vi "固定站CODMn测量流程.vi"(11 "控制命令":u16(ring)=1 items=["启动测量"=1, "标样核查"=2, "零点核查"=3, "跨度核查"=4, "空白测试"=5, "平行样测试"=6, "加标回收"=7, "空白校准"=8, "标样校准"=9, "初始化（清洗）"=10, "停止测试"=11, "仪器重启"=12, "校时"=13, "模式设置"=14, "测量间隔设置"=15, "调试"=22, "填充管路"=30, "清洗管路"=31, "清洗反应杯"=32]) -> ()   [LabVIEW 2016, in "斯坦道CODMn新电路板.lvlib"]
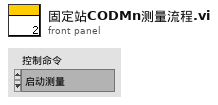
[diagram p1: front panel]
types:
  T1 = cluster{"仪器":enum16{"", "氨氮", "总磷", "总氮", "CODMn", "CODCr"}, "启动命令":enum16{"启动水样流程", "启动加标流程", "排液", "停止", "柱塞泵启动"}}
  T2 = cluster{"时间标识":timestamp, "设备":string, "日志信息":string, "备注":string}
  T3 = cluster{"站号":u16, "量程切换":enum32{"H", "L", "AUTO"}, "控制命令":u16, "模式设置":enum16{"待机", "连续模式", "周期模式", "定点模式", "受控模式", "手动模式"}, "测量间隔":u16}
  T4 = cluster{"系统时间":timestamp, "工作状态":u16, "测量模式":enum16{"待机", "连续模式", "周期模式", "定点模式", "受控模式", "手动模式"}, "告警代码":u16, "故障代码":u16, "日志代码":u16, "软件版本":u16, "A":sgl, "B":sgl, "K":sgl, "当前滴定数":sgl, "T":sgl, "H":sgl, "id":u16, "flowid":u16, "量程":u16, "加热实时温度":sgl, "当前ORP值":sgl, "运行时间":sgl, "当前步骤剩余时间":sgl, "结束滴定数":sgl, "注射泵保温温度":sgl}
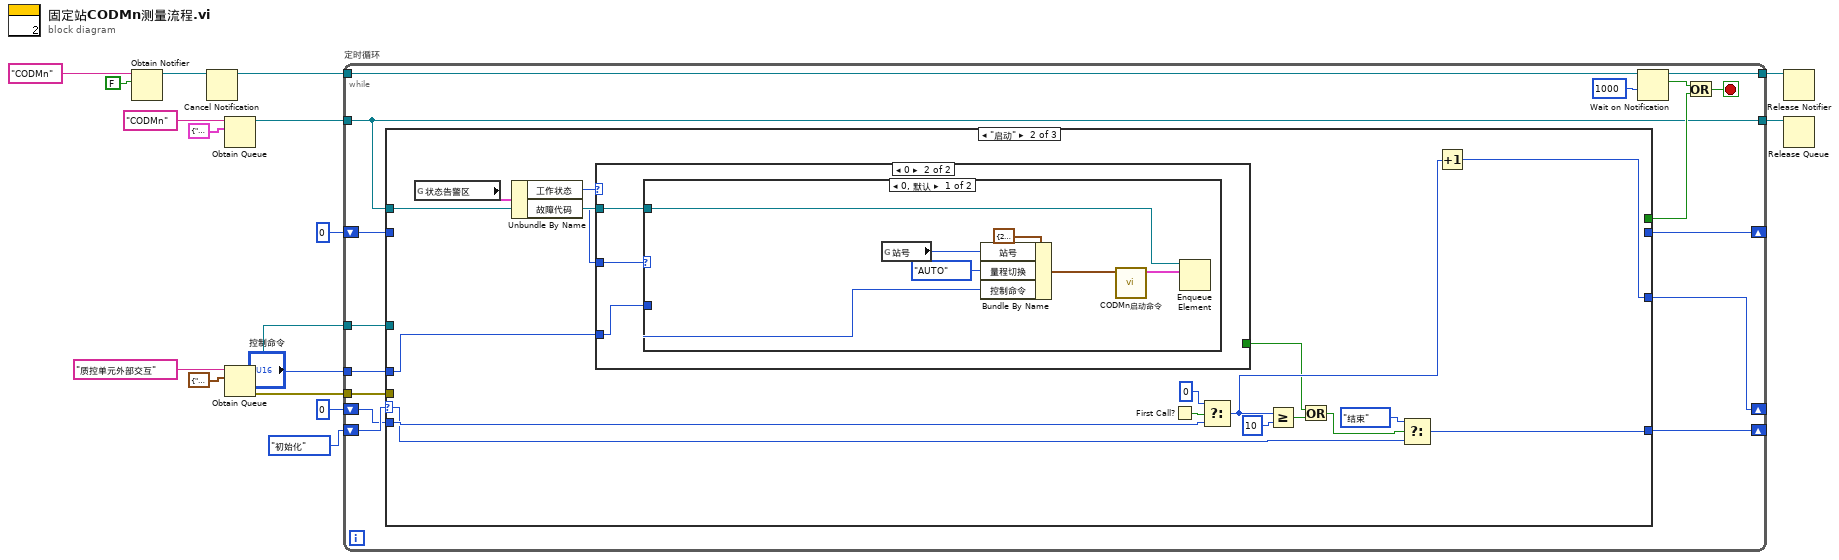
[diagram p0: block diagram]
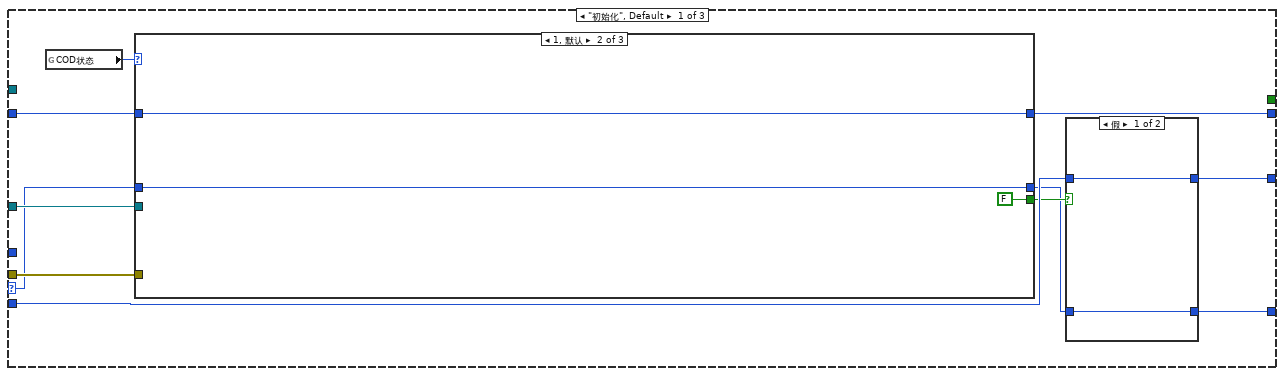
[diagram p2: hidden frame]
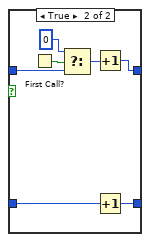
[diagram p3: hidden frame]
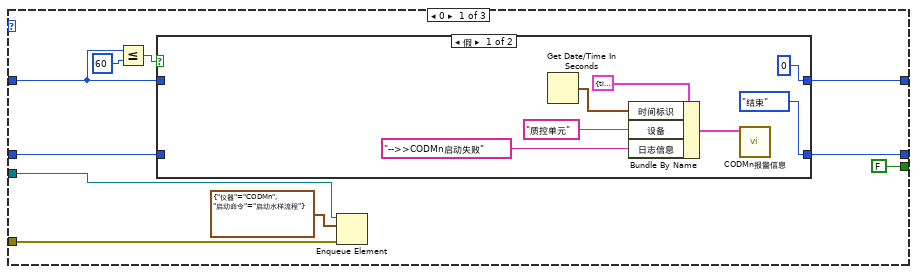
[diagram p4: hidden frame]
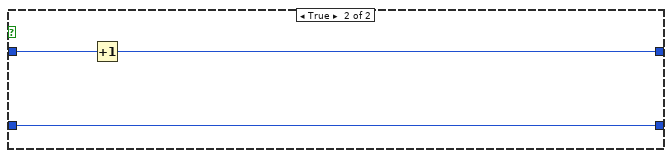
[diagram p5: hidden frame]
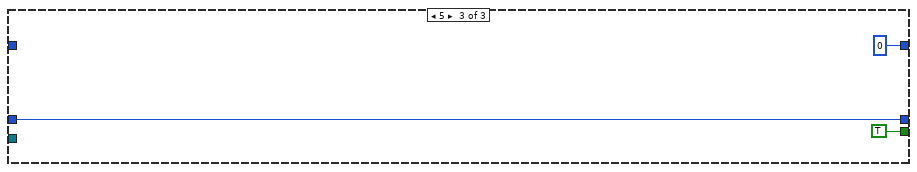
[diagram p6: hidden frame]
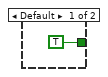
[diagram p7: hidden frame]
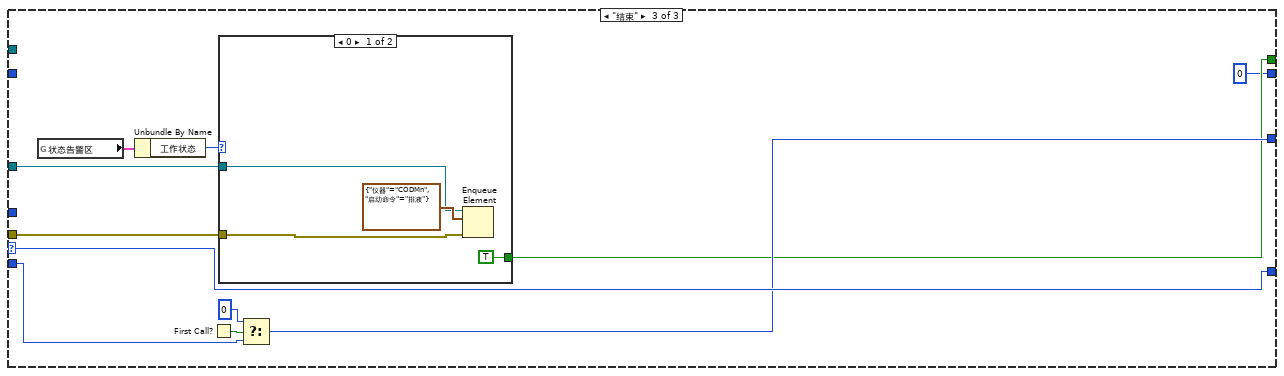
[diagram p9: hidden frame]
diagram:
  n1 = Obtain Notifier(name (unnamed)="CODMn" ("名称（未命名）"), notification data type=FALSE) -> (notifier out=w12:refnum<notifier>)  [unwired: 2 in, 2 out]
  n2 = Cancel Notification(0:w12) -> (8:w11:refnum<notifier>)  [unwired: 1 in, 2 out]
  n3 = Obtain Queue(name (unnamed)="CODMn" ("名称（未命名）"), element data type=cluster{"命令":string, "data":variant} {"命令"="", "data"=variant}) -> (queue out=w15:refnum<queue>)  [unwired: 3 in, 2 out]
  n4 = Obtain Queue(name (unnamed)="质控单元外部交互" ("名称（未命名）"), element data type=T1 {"仪器"=enum."氨氮", "启动命令"=enum."启动水样流程"} ("元素")) -> (queue out=w4:refnum<queue>, error out=w3:errorcluster)  [unwired: 3 in, 1 out]
  n5 = while "定时循环" {
    tunnel: w15 -> [w22]
    tunnel: w11 -> [w33]
    tunnel: "控制命令" -> [w28]
    shift-right: [w27] -> _
    shift-left: enum16{"初始化", "启动", "结束"}."初始化" -> [w29]
    shift-right: [w25] -> _
    shift-left: 0 -> [w26]
    tunnel: [w23] -> w7
    tunnel: [w22] -> w8
    tunnel: w4 -> [w21]
    tunnel: w3 -> [w20]
    shift-right: [w18] -> _
    shift-left: 0 -> [w19]
    stop <- w30 stop-if-true
    n6 = case shown="\"启动\"" w29 {
      selector: w29 -> [w35 w85 w118]
      tunnel: w28 -> [_ w96 _]
      tunnel: w22 -> [_ w95 _]
      tunnel: [w44 w86 w118] -> w27
      tunnel: w26 -> [w43 w90 w115]
      tunnel: [w42 w89 w114] -> w25
      tunnel: [_ _ w109] -> w24
      tunnel: w21 -> [w39 _ w113]
      tunnel: w20 -> [w38 _ w112]
      tunnel: w19 -> [w37 _ _]
      tunnel: [w36 _ 0] -> w18
      frame "初始化", Default {
        n7 = global read "VARCODMn全局变量.vi" "COD状态"() -> (w40:u16)
        n8 = case shown="1, 默认" w40 {
          tunnel: [FALSE ("s") FALSE ("s") TRUE ("s")] -> w41
          tunnel: w39 -> [w62 _ _]
          tunnel: w38 -> [w61 _ _]
          tunnel: w37 -> [w59 w74 _]
          tunnel: [w56 w74 0] -> w36
          tunnel: w35 -> [w55 w75 w78]
          tunnel: [w54 w75 w78] -> w34
          frame 0 {
            n9 = Less Or Equal?(x=w59, y=60) -> (x <= y?=w57:bool)
            n10 = case shown="假" w57 {
              tunnel: w59 -> [_ w73]
              tunnel: [0 w72] -> w56
              tunnel: w55 -> [_ w71]
              tunnel: [enum16{"初始化", "启动", "结束"}."结束" w71] -> w54
              frame False {
                n11 = Get Date/Time In Seconds() -> (seconds since 1Jan1904=w66:timestamp)
                n12 = Bundle By Name(cluster=T2 {"时间标识"=timestamp(0 s since 1904-01-01), "设备"="", "日志信息"="", "备注"=""} ("data in"), "时间标识"=w66, "设备"="质控单元", "日志信息"="-->>CODMn启动失败") -> (w64:T2)
                n13 = call "CODMn报警信息.vi"("data in"=w64) -> ()  [unwired: 10 in, 1 out]
              }
              frame True {
                n14 = Increment(x=w73) -> (x+1=w72:i32)
              }
            }
            n15 = Enqueue Element(queue=w62, element=T1 {"仪器"=enum."CODMn", "启动命令"=enum."启动水样流程"} ("元素"), error in (no error)=w61) -> ()  [unwired: 1 in, 3 out]
          }
          frame 1, Default {
          }
          frame 5 {
          }
        }
        n16 = case shown="假" w41 {
          tunnel: w34 -> [w46 w53]
          tunnel: [w46 w52] -> w44
          tunnel: w43 -> [w45 w50]
          tunnel: [w45 w47] -> w42
          frame False {
          }
          frame True {
            n17 = First Call?() -> (First Call?: T/F=w51:bool)
            n18 = Select(t=0, s=w51, f=w50) -> (s? t:f=w48:i32)
            n19 = Increment(x=w48) -> (x+1=w47:i32)
            n20 = Increment(x=w53) -> (x+1=w52:enum16{"初始化", "启动", "结束"})
          }
        }
      }
      frame "启动" {
        n21 = global read "VARCODMn全局变量.vi" "状态告警区"() -> (w94:T4)
        n22 = Unbundle By Name(w94) -> ("工作状态"=w93:u16, "故障代码"=w80:u16)
        n23 = case shown="0" w93 {
          tunnel: w96 -> [_ w99]
          tunnel: w95 -> [_ w100]
          tunnel: [TRUE _] -> w81
          tunnel: w80 -> [_ w98]
          frame Default {
          }
          frame 0 {
            n24 = case shown="0, 默认" w98 {
              tunnel: w100 -> [w106 _]
              tunnel: w99 -> [w105 _]
              frame 0, Default {
                n25 = global read "CODMn断电保存全局变量.vi" "站号"() -> (w104:u16)
                n26 = Bundle By Name(cluster=T3 {"站号"=21, "量程切换"=enum."AUTO", "控制命令"=0, "模式设置"=enum."受控模式", "测量间隔"=0} ("参数"), "站号"=w104, "量程切换"=enum32{"H", "L", "AUTO"}."AUTO", "控制命令"=w105) -> (w101:T3)
                n27 = call "CODMn启动命令.vi"("参数"=w101) -> ("启动命令"=w107:cluster{"命令":string, "data":variant})  [unwired: 10 in]
                n28 = Enqueue Element(queue=w106, element=w107) -> ()  [unwired: 2 in, 3 out]
              }
              frame 2 {
                # "加热故障"
              }
            }
          }
        }
        n29 = First Call?() -> (First Call?: T/F=w92:bool)
        n30 = Select(t=0, s=w92, f=w90) -> (s? t:f=w88:i32)
        n31 = Greater Or Equal?(x=w88, y=10) -> (x >= y?=w84:bool)
        n32 = Or(x=w81, y=w84) -> (x .or. y?=w82:bool)
        n33 = Select(t=enum16{"初始化", "启动", "结束"}."结束", s=w82, f=w85) -> (s? t:f=w86:enum16{"初始化", "启动", "结束"})
        n34 = Increment(x=w88) -> (x+1=w89:i32)
      }
      frame "结束" {
        n35 = global read "VARCODMn全局变量.vi" "状态告警区"() -> (w111:T4)
        n36 = Unbundle By Name(w111) -> ("工作状态"=w110:u16)
        n37 = First Call?() -> (First Call?: T/F=w117:bool)
        n38 = case shown="0" w110 {
          tunnel: w113 -> [w121 _]
          tunnel: w112 -> [w120 _]
          tunnel: [TRUE _] -> w109
          frame 0 {
            n39 = Enqueue Element(queue=w121, element=T1 {"仪器"=enum."CODMn", "启动命令"=enum."排液"} ("元素"), error in (no error)=w120) -> ()  [unwired: 1 in, 3 out]
          }
          frame 1, Default {
          }
        }
        n40 = Select(t=0, s=w117, f=w115) -> (s? t:f=w114:i32)
      }
    }
    n41 = Wait on Notification(notifier=w33, timeout in ms (-1)=1000 ("超时毫秒(-1)")) -> (notifier out=w23:refnum<notifier>, notification=w31:bool)  [unwired: 2 in, 2 out]
    n42 = Or(x=w31, y=w24) -> (x .or. y?=w30:bool)
  }
  n43 = Release Notifier(notifier=w7) -> ()  [unwired: 2 in, 3 out]
  n44 = Release Queue(queue=w8) -> ()  [unwired: 2 in, 3 out]
